vi "PI Receive String.vi"(0 "System no.":i32=1 min=1 step=1, 3 "Strip spaces?":bool, 5 "error in":errorcluster) -> (14 "String read":string, 15 "bytes read":u16, 19 "error out":errorcluster)   [LabVIEW 2026]
doc: "Read string from selected system."
uses:
  Available interfaces.ctl
  Available DLLs.ctl
  Available DLL interfaces.ctl
  Termination character.ctl
  Syntax.ctl
  Global1.vi
panel:
  out "Logging mode":bool
  out "Syntax":T1
  out "Termination character":T2
  out "VISA resource name":refnum<visa-resource-name>
  out "TCP/IP\nConfiguration":T3={"Host address/name"="localhost", "Port"=0, "Board"=4}
  out "DLL Interface Configuration":T6 {"DLL for Device" items=["C-843", "C-844", "E-710", "C-843.PM", "C-865", "E-761", "Mercury", "E-755", "E-753", "C-866", "E-712", "E-725", "E-861", "C-867", "E-517", "E-816", "E-709", "PI_GCS2_DLL", "HydraPollux"]; "DLL Interface" items=["RS232", "GPIB", "Board", "TCP-IP", "USB", "RS232_DC"]}
  out "Interface configuration":T8={"RS232 Portnumber"=0, "Timeout"=5000, "RS232 baud rate"=57600, "Interface"=0, "GPIB Bus"=0, "GPIB address"=4, "GPIB Mode"=0} {"Interface" items=["RS232", "GPIB", "DLL", "TCP-IP", "USB", "Analog"]; "RS232 Portnumber" items=["COM1", "COM2", "COM3", "COM4", "COM5", "COM6", "COM7", "COM8", "COM9", "COM10", "COM11", "COM12", "COM13", "COM14", "COM15", "COM16", "COM17", "COM18", "COM19", "COM20", "COM21", "COM22", "COM23", "COM24", "COM25", "COM26", "COM27", "COM28", "COM29", "COM30"]}
  # "This vi receives a string via the selected interface."
  # "Communication setup indicators (for troubleshooting):"
  # "TCP/IP:"
  # "DLL:"
  # "General:"
  # "RS232:"
  # "GPIB:"
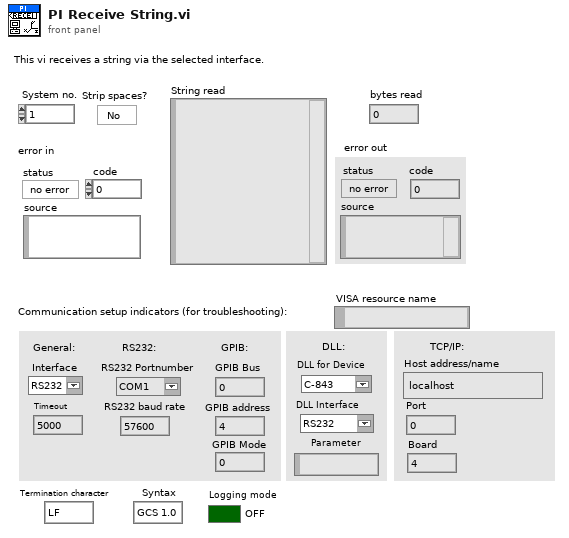
[diagram p1: front panel]
types:
  T1 = typedef "Syntax.ctl" = enum16{"GCS 1.0", "GCS 2.0", "GCS 3.0"}
  T2 = typedef "Termination character.ctl" = enum16{"LF", "CR", "LFCR", "CRLF"}
  T3 = cluster{"Host address/name":string, "Port":i32, "Board":i32}
  T4 = typedef "Available DLLs.ctl" = u16
  T5 = typedef "Available DLL interfaces.ctl" = u16
  T6 = cluster{"DLL for Device":T4, "DLL Interface":T5, "Parameter":string}
  T7 = typedef "Available interfaces.ctl" = u16
  T8 = cluster{"RS232 Portnumber":i32, "Timeout":i32, "RS232 baud rate":u32, "Interface":T7, "GPIB Bus":i32, "GPIB address":i32, "GPIB Mode":i32}
  T9 = cluster{"DLL for Device":T4, "DLL Interface":T5, "Parameter":string}[]
  T10 = cluster{"RS232 Portnumber":i32, "Timeout":i32, "RS232 Baud rate":u32, "Interface":T7, "GPIB Bus":i32, "GPIB Address":i32, "GPIB Mode":i32}[]
  T11 = cluster{"Host address/name":string, "Port":i32, "Board":i32}[]
  T12 = cluster{"RS232 Portnumber":i32, "Timeout":i32, "RS232 Baud rate":u32, "Interface":T7, "GPIB Bus":i32, "GPIB Address":i32, "GPIB Mode":i32}
  T13 = enum16{"C844_IsDLLAvailable", "C844_ConnectRS232", "C844_ConnectNIgpib", "C844_IsConnected", "C844_CloseConnection", "C844_GcsCommandset", "C844_GetError", "C844_GcsGetAnswerSize", "C844_GcsGetAnswer", "C843_IsDLLAvailable", "C843_Connect", "C843_IsConnected", "C843_CloseConnection", "C843_GcsCommandset", "C843_GetError", "C843_GcsGetAnswerSize", "C843_GcsGetAnswer", "E710_IsDLLAvailable", "E710_ConnectRS232", "E710_ConnectNIgpib", "E710_IsConnected", "E710_CloseConnection", "E710_GcsCommandset", "E710_GetError", "E710_GcsGetAnswerSize", "E710_GcsGetAnswer", "C843_PM_IsDLLAvailable", "C843_PM_Connect", "C843_PM_IsConnected", "C843_PM_CloseConnection", "C843_PM_GcsCommandset", "C843_PM_GetError", "C843_PM_GcsGetAnswerSize", "C843_PM_GcsGetAnswer", "C843_PM_GetCurrentBoardID", "C843_GetCurrentBoardID", "C865_IsDLLAvailable", "C865_ConnectRS232", "C865_IsConnected", "C865_CloseConnection", "C865_GcsCommandset", "C865_GetError", "C865_GcsGetAnswerSize", "C865_GcsGetAnswer", "C865_GetCurrentInterfaceID", "E761_ConnectPciBoard", "DefineSystem", "CloseConnection", "IsConnected", "ConnectRS232", "ConnectNIgpib", "ConnectPciBoard", "ConnectTCPIP", "GetError", "GcsCommandset", "GCSGetAnswerSize", "GcsGetAnswer", "CloseDaisyChain", "OpenRS232DaisyChain", "ConnectDaisyChainDevice", "ConnectUSB", "ListUSB", "OpenUSBDaisyChain", "OpenTCPIPDaisyChain"}
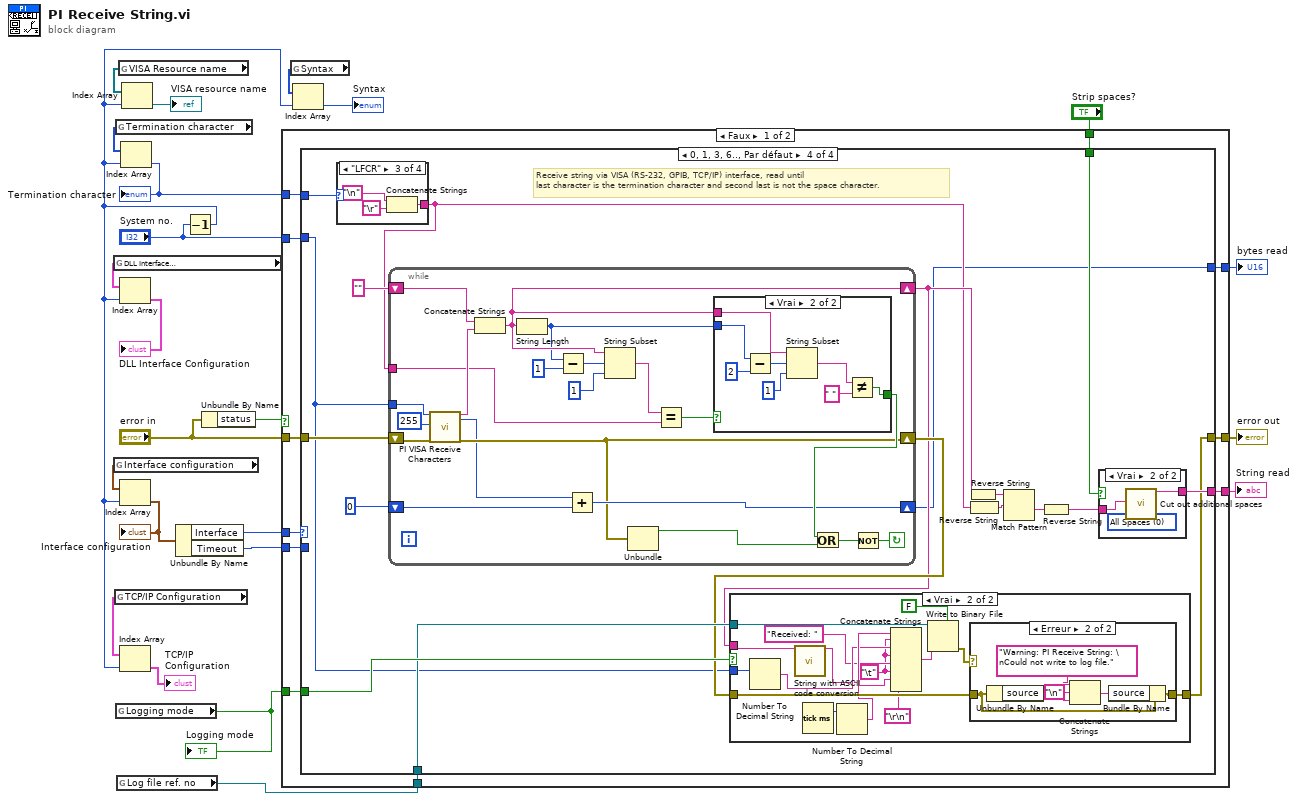
[diagram p0: block diagram]
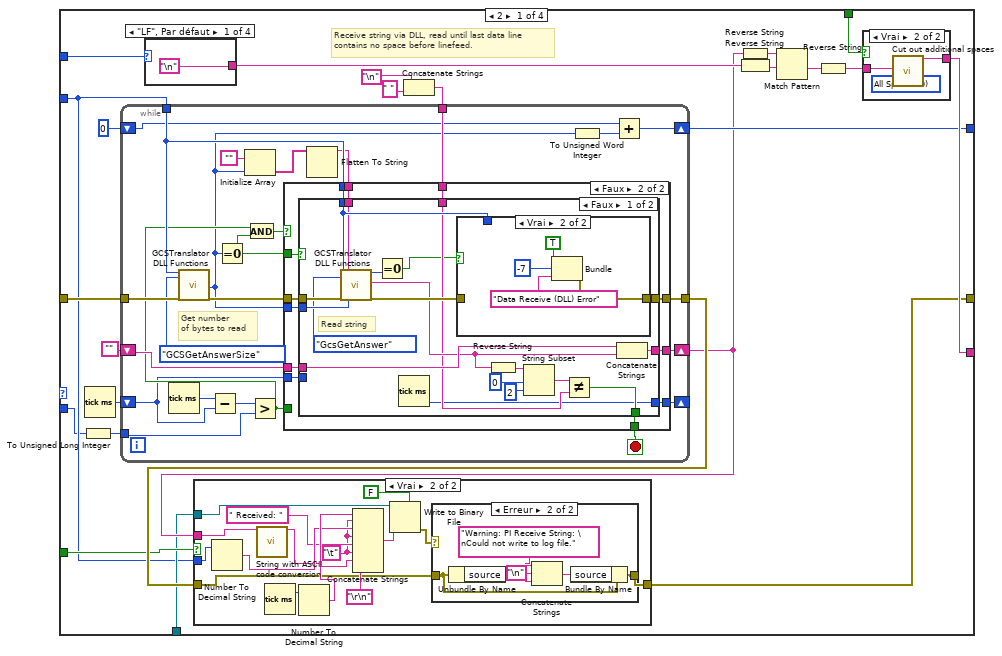
[diagram p2: hidden frame]
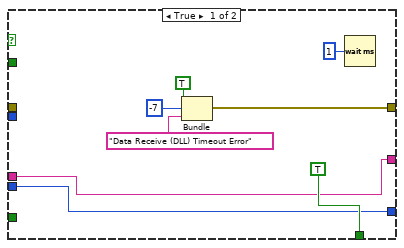
[diagram p5: hidden frame]
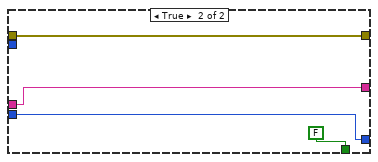
[diagram p7: hidden frame]
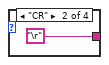
[diagram p8: hidden frame]
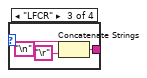
[diagram p9: hidden frame]
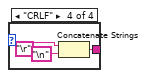
[diagram p10: hidden frame]
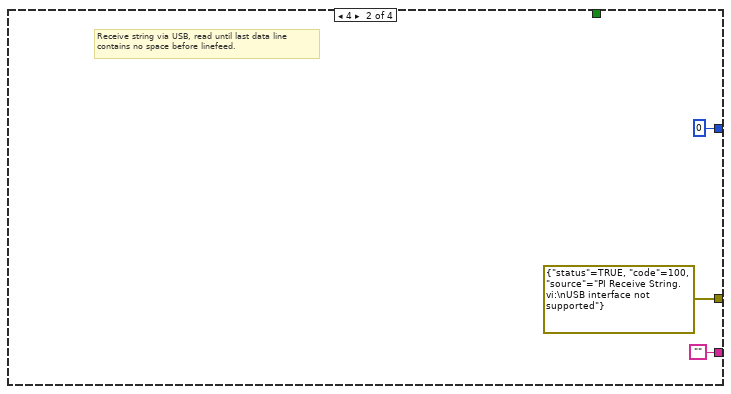
[diagram p12: hidden frame]
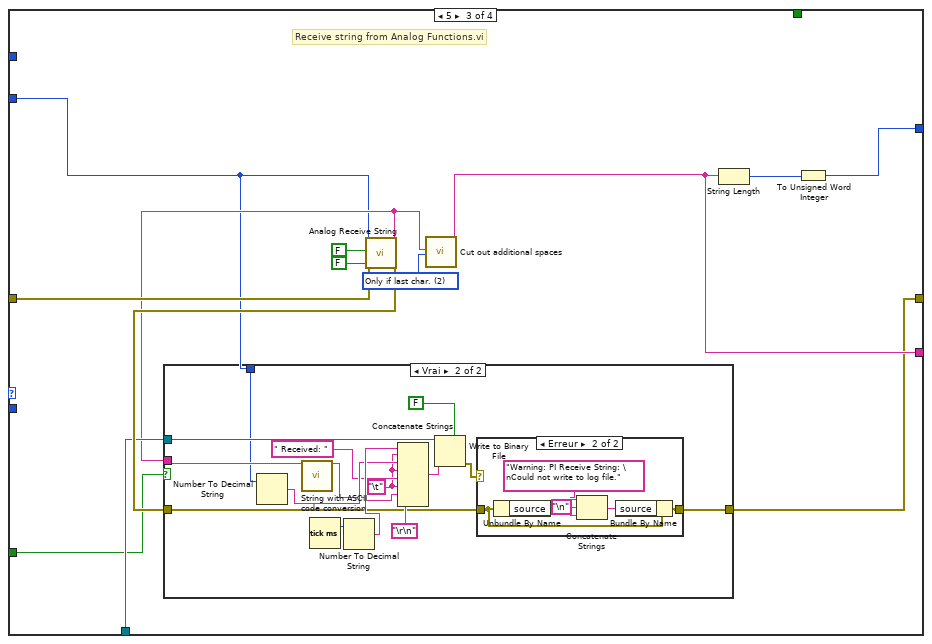
[diagram p13: hidden frame]
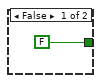
[diagram p16: hidden frame]
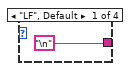
[diagram p20: hidden frame]
diagram:
  n1 = global read "Global1.vi" "DLL Interface\nConfiguration"() -> (w16:T9)
  n2 = global read "Global1.vi" "Interface configuration"() -> (w21:T10)
  n3 = global read "Global1.vi" "TCP/IP Configuration"() -> (w11:T11)
  n4 = global read "Global1.vi" "Termination character"() -> (w9:T2[])
  n5 = global read "Global1.vi" "Logging mode"() -> (w2:bool)
  "Logging mode" <- w2
  n6 = global read "Global1.vi" "Log file ref. no"() -> (w1:refnum<file>)
  n7 = global read "Global1.vi" "VISA Resource name"() -> (w13:refnum<visa-resource-name>[])
  n8 = Decrement(x="System no.") -> (x-1=w3:i32)
  n9 = Index Array(array=w16, index=w3) -> (element=→"DLL Interface Configuration":T6)
  n10 = Index Array(array=w21, index=w3) -> (element=w14:T12)
  "Interface configuration" <- w14
  n11 = Index Array(array=w11, index=w3) -> (element=→"TCP/IP\nConfiguration":T3)
  n12 = Index Array(array=w9, index=w3) -> (element=w8:T2)
  "Termination character" <- w8
  n13 = Index Array(array=w13, index=w3) -> (element=→"VISA resource name":refnum<visa-resource-name>)
  n14 = Unbundle By Name(w14) -> ("Interface"=w17:T7, "Timeout"=w4:i32)
  n15 = Unbundle By Name("error in") -> ("status"=w18:bool)
  n16 = case shown="Faux" w18 {
    tunnel: [w35 "" ("String read")] -> w24
    tunnel: "error in" -> [w34 w289]
    tunnel: w17 -> [w33 _]
    tunnel: [w32 u16 0 ("Bytes read")] -> w23
    tunnel: [w31 w289] -> w22
    tunnel: "System no." -> [w30 _]
    tunnel: w8 -> [w29 _]
    tunnel: "Strip spaces?" -> [w28 _]
    tunnel: w4 -> [w27 _]
    tunnel: w2 -> [w26 _]
    tunnel: w1 -> [w25 _]
    frame False {
      n17 = case shown="0, 1, 3, 6.., Par défaut" w33 {
        tunnel: [w58 "" ("String out") w181 w218] -> w35
        tunnel: w34 -> [w59 _ w178 w213]
        tunnel: [w50 u16 0 w170 w207] -> w32
        tunnel: [w39 errorcluster {"status"=TRUE, "code"=100, "source"="PI Receive String.vi:\nUSB interface not supported"} w176 w214] -> w31
        tunnel: w30 -> [w38 _ w172 w208]
        tunnel: w29 -> [w53 _ _ w223]
        tunnel: w28 -> [w57 _ _ w217]
        tunnel: w27 -> [w36 _ _ _]
        tunnel: w26 -> [w41 _ w174 w216]
        tunnel: w25 -> [w40 _ w175 w215]
        frame 2 {
          # "Receive string via DLL, read until last data line\ncontains no space before linefeed."
          n18 = To Unsigned Long Integer(number=w36) -> (unsigned 32bit integer=w37:u32)
          n19 = Tick Count (ms)() -> (millisecond timer value=w44:u32)
          n20 = case shown="\"LF\", Par défaut" w53 {
            tunnel: ["\n" "\r" w157 w162] -> w52
            frame "LF", Default {
            }
            frame "CR" {
            }
            frame "LFCR" {
              n21 = Concatenate Strings("\n", "\r") -> (w157:string)
            }
            frame "CRLF" {
              n22 = Concatenate Strings("\r", "\n") -> (w162:string)
            }
          }
          n23 = Concatenate Strings("\n", " " ("string")) -> (w47:string)
          n24 = while {
            tunnel: w59 -> [w106]
            tunnel: [w105] -> w43
            tunnel: w38 -> [w104]
            shift-right: [w98] -> w42
            shift-left: "" -> [w97]
            tunnel: w47 -> [w96]
            tunnel: w37 -> [w83]
            shift-right: [w89] -> _
            shift-left: w44 -> [w88]
            shift-right: [w99] -> w50
            shift-left: u16 0 -> [w86]
            stop <- w95 stop-if-true
            # "Get number\nof bytes to read"
            n25 = Tick Count (ms)() -> (millisecond timer value=w93:u32)
            n26 = call "GCSTranslator DLL Functions.vi"("System no."=w104, "Function"=T13."GCSGetAnswerSize", "error in"=w106) -> ("Numerical output"=w84:i32, "error out"=w100:errorcluster)  [unwired: 4 in, 11 out]
            n27 = Subtract(x=w93, y=w88) -> (x-y=w92:u32)
            n28 = Equal To 0?(x=w84) -> (x = 0?=w90:bool)
            n29 = Initialize Array("", w84) -> (w102:string[])
            n30 = Greater?(x=w92, y=w83) -> (0:w91:bool)
            n31 = And(x=w91, y=w90) -> (x .and. y?=w94:bool)
            n32 = Flatten To String(anything=w102) -> (data string=w101:string)  [unwired: 1 in, 4 out]
            n33 = case shown="Faux" w94 {
              tunnel: [w114 w126] -> w105
              tunnel: w104 -> [_ w125]
              tunnel: w101 -> [_ w124]
              tunnel: w100 -> [_ w123]
              tunnel: w84 -> [_ w122]
              tunnel: [w111 w121] -> w98
              tunnel: w97 -> [w111 w120]
              tunnel: w96 -> [_ w119]
              tunnel: [TRUE w118] -> w95
              tunnel: w91 -> [_ _]
              tunnel: w90 -> [_ w116]
              tunnel: [w110 w117] -> w89
              tunnel: w88 -> [w110 w115]
              frame True {
                n34 = Bundle(TRUE, -7, "Data Receive (DLL) Timeout Error") -> (w114:errorcluster)  [unwired: 1 out]
                n35 = Wait (ms)(milliseconds to wait=u32 1) -> ()  [unwired: 1 out]
              }
              frame False {
                n36 = case shown="Faux" w116 {
                  tunnel: [w145 w154] -> w126
                  tunnel: w125 -> [w144 _]
                  tunnel: w124 -> [w143 _]
                  tunnel: w123 -> [w142 w154]
                  tunnel: w122 -> [w139 _]
                  tunnel: [w138 w153] -> w121
                  tunnel: w120 -> [w137 w153]
                  tunnel: w119 -> [w132 _]
                  tunnel: [w131 FALSE] -> w118
                  tunnel: [w128 w152] -> w117
                  tunnel: w115 -> [_ w152]
                  frame False {
                    # "Read string"
                    n37 = call "GCSTranslator DLL Functions.vi"("System no."=w144, "Function"=T13."GcsGetAnswer", "error in"=w142, "String buffer"=w143, "Numerical input"=w139) -> ("DLL I32 Return value"=w141:i32, "String output"=w136:string, "error out"=w140:errorcluster)  [unwired: 2 in, 10 out]
                    n38 = Equal To 0?(x=w141) -> (x = 0?=w129:bool)
                    n39 = Tick Count (ms)() -> (millisecond timer value=w128:u32)
                    n40 = case shown="Vrai" w129 {
                      tunnel: [w146 w148] -> w145
                      tunnel: w144 -> [_ _]
                      tunnel: w140 -> [w146 _]
                      frame False {
                        # "no error"
                      }
                      frame True {
                        n41 = Bundle(TRUE, -7, "Data Receive (DLL) Error") -> (w148:errorcluster)  [unwired: 1 out]
                      }
                    }
                    n42 = Reverse String(1:w136) -> (0:w135:string)
                    n43 = String Subset(string=w135, offset (0)=0, length (rest)=2 ("length (rest)")) -> (substring=w133:string)
                    n44 = Not Equal?(x=w133, y=w132) -> (x != y?=w131:bool)
                    n45 = Concatenate Strings(w137, w136) -> (w138:string)
                  }
                  frame True {
                  }
                }
              }
            }
            n46 = To Unsigned Word Integer(number=w84) -> (unsigned 16bit integer=w85:u16)
            n47 = Add(x=w86, y=w85) -> (x+y=w99:u16)
          }
          n48 = case shown="Vrai" w41 {
            tunnel: w40 -> [_ w64]
            tunnel: w42 -> [_ w63]
            tunnel: w43 -> [w60 w65]
            tunnel: [w60 w66] -> w39
            tunnel: w38 -> [_ w62]
            frame False {
            }
            frame True {
              w69 = "\t"
              n49 = Number To Decimal String(number=w62) -> (decimal integer string=w71:string)  [unwired: 1 out]
              n50 = call "String with ASCII code conversion.vi"("Input string"=w63) -> ("Output string"=w68:string)  [unwired: 18 out]
              n51 = Tick Count (ms)() -> (millisecond timer value=w73:u32)
              n52 = Number To Decimal String(number=w73) -> (decimal integer string=w72:string)  [unwired: 1 out]
              n53 = Concatenate Strings(w72, w69, w71, w69, " Received: " ("string"), w69, w68, "\r\n") -> (w75:string)
              n54 = Write to Binary File(file (use dialog)=w64, data=w75, 5:FALSE ("prepend array or string size? (T)")) -> (error out=w74:errorcluster)  [unwired: 1 in, 4 out]
              n55 = case shown="Erreur" w74 {
                tunnel: w65 -> [w76 w82]
                tunnel: [w76 w78] -> w66
                frame No Error {
                }
                frame Error {
                  n56 = Unbundle By Name(w82) -> ("source"=w81:string)
                  n57 = Concatenate Strings(w81, "\n" ("string"), "Warning: PI Receive String: \nCould not write to log file." ("source")) -> (w77:string)
                  n58 = Bundle By Name(cluster=w82, "source"=w77) -> (w78:errorcluster)
                }
              }
            }
          }
          n59 = Reverse String(1:w42) -> (0:w55:string)
          n60 = Reverse String(1:w52) -> (0:w54:string)
          n61 = Match Pattern(string=w55, regular expression=w54) -> (after substring=w56:string)  [unwired: 4 out]
          n62 = Reverse String(1:w56) -> (0:w51:string)
          n63 = case shown="Vrai" w57 {
            tunnel: w51 -> [w163 w166]
            tunnel: [w163 w165] -> w58
            frame False {
            }
            frame True {
              w164 = u16 0 items=["All Spaces", "Only if 1st char.", "Only if last char.", "Only if near \"=\"", "Only if 1st or last char.", "Only multiple"] ("Mode")
              n64 = call "Cut out additional spaces.vi"("String"=w166, "Mode"=w164) -> ("String out"=w165:string)  [unwired: 17 out]
            }
          }
        }
        frame 4 {
          # "Receive string via USB, read until last data line\ncontains no space before linefeed."
        }
        frame 5 {
          w182 = u16 2 items=["All Spaces", "Only if 1st char.", "Only if last char.", "Only if near \"=\"", "Only if 1st or last char.", "Only multiple"] ("Mode")
          # "Receive string from Analog Functions.vi"
          n65 = call "Analog Receive String.vi"("System no."=w172, "Read/Write (T)"=FALSE, "Ini"=FALSE, "error in"=w178) -> ("String out"=w173:string, "error out"=w177:errorcluster)  [unwired: 1 in, 13 out]
          n66 = case shown="Vrai" w174 {
            tunnel: w175 -> [_ w189]
            tunnel: w173 -> [_ w188]
            tunnel: w177 -> [w183 w187]
            tunnel: [w183 w186] -> w176
            tunnel: w172 -> [_ w185]
            frame False {
            }
            frame True {
              w192 = "\t"
              n67 = Number To Decimal String(number=w185) -> (decimal integer string=w194:string)  [unwired: 1 out]
              n68 = call "String with ASCII code conversion.vi"("Input string"=w188) -> ("Output string"=w191:string)  [unwired: 18 out]
              n69 = Tick Count (ms)() -> (millisecond timer value=w196:u32)
              n70 = Number To Decimal String(number=w196) -> (decimal integer string=w195:string)  [unwired: 1 out]
              n71 = Concatenate Strings(w195, w192, w194, w192, " Received: " ("string"), w192, w191, "\r\n") -> (w198:string)
              n72 = Write to Binary File(file (use dialog)=w189, data=w198, 5:FALSE ("prepend array or string size? (T)")) -> (error out=w197:errorcluster)  [unwired: 1 in, 4 out]
              n73 = case shown="Erreur" w197 {
                tunnel: w187 -> [w199 w205]
                tunnel: [w199 w201] -> w186
                frame No Error {
                }
                frame Error {
                  n74 = Unbundle By Name(w205) -> ("source"=w204:string)
                  n75 = Concatenate Strings(w204, "\n" ("string"), "Warning: PI Receive String: \nCould not write to log file." ("source")) -> (w200:string)
                  n76 = Bundle By Name(cluster=w205, "source"=w200) -> (w201:errorcluster)
                }
              }
            }
          }
          n77 = call "Cut out additional spaces.vi"("String"=w173, "Mode"=w182) -> ("String out"=w181:string)  [unwired: 17 out]
          n78 = String Length(string=w181) -> (length=w171:i32)
          n79 = To Unsigned Word Integer(number=w171) -> (unsigned 16bit integer=w170:u16)
        }
        frame 0, 1, 3, 6.., Default {
          # "Receive string via VISA (RS-232, GPIB, TCP/IP) interface, read until \nlast character is the termination character and second last is not the space character."
          n80 = case shown="\"LFCR\"" w223 {
            tunnel: ["\n" "\r" w283 w288] -> w209
            frame "LF", Default {
            }
            frame "CR" {
            }
            frame "LFCR" {
              n81 = Concatenate Strings("\n", "\r") -> (w283:string)
            }
            frame "CRLF" {
              n82 = Concatenate Strings("\r", "\n") -> (w288:string)
            }
          }
          n83 = while {
            shift-left: w213 -> [w237]
            shift-right: [w236] -> w212
            tunnel: w208 -> [w235]
            shift-left: u16 0 -> [w239]
            shift-right: [w238] -> w207
            shift-left: "" -> [w244]
            shift-right: [w225] -> w211
            tunnel: w209 -> [w227]
            stop <- w241 continue-if-true
            n84 = call "PI VISA Receive Characters.vi"("System no."=w235, "Bytes to read"=u16 255, "error in"=w237) -> ("String read"=w232:string, "Bytes read"=w233:u16, "error out"=w236:errorcluster)  [unwired: 14 out]
            n85 = Concatenate Strings(w244, w232) -> (w225:string)
            n86 = String Length(string=w225) -> (length=w224:i32)
            n87 = Subtract(x=w224, y=1) -> (x-y=w230:i32)
            n88 = Add(x=w233, y=w239) -> (x+y=w238:u16)
            n89 = String Subset(string=w225, offset (0)=w230, length (rest)=1 ("length (rest)")) -> (substring=w228:string)
            n90 = Unbundle(w236) -> ("status"=w243:bool)  [unwired: 2 out]
            n91 = Equal?(x=w228, y=w227) -> (x = y?=w226:bool)
            n92 = case shown="Vrai" w226 {
              tunnel: [FALSE w252] -> w240
              tunnel: w225 -> [_ w250]
              tunnel: w224 -> [_ w246]
              frame False {
              }
              frame True {
                n93 = Subtract(x=w246, y=2) -> (x-y=w247:i32)
                n94 = String Subset(string=w250, offset (0)=w247, length (rest)=1 ("length (rest)")) -> (substring=w249:string)
                n95 = Not Equal?(x=w249, y=" ") -> (x != y?=w252:bool)
              }
            }
            n96 = Or(x=w240, y=w243) -> (x .or. y?=w242:bool)
            n97 = Not(x=w242) -> (.not. x?=w241:bool)
          }
          n98 = case shown="Vrai" w216 {
            tunnel: w215 -> [_ w269]
            tunnel: w211 -> [_ w264]
            tunnel: w212 -> [w254 w266]
            tunnel: [w254 w265] -> w214
            tunnel: w208 -> [_ w263]
            frame False {
            }
            frame True {
              w258 = "\t"
              n99 = Number To Decimal String(number=w263) -> (decimal integer string=w260:string)  [unwired: 1 out]
              n100 = call "String with ASCII code conversion.vi"("Input string"=w264) -> ("Output string"=w257:string)  [unwired: 18 out]
              n101 = Tick Count (ms)() -> (millisecond timer value=w262:u32)
              n102 = Number To Decimal String(number=w262) -> (decimal integer string=w261:string)  [unwired: 1 out]
              n103 = Concatenate Strings(w261, w258, w260, w258, "Received: " ("string"), w258, w257, "\r\n") -> (w268:string)
              n104 = Write to Binary File(file (use dialog)=w269, data=w268, 5:FALSE ("prepend array or string size? (T)")) -> (error out=w267:errorcluster)  [unwired: 1 in, 4 out]
              n105 = case shown="Erreur" w267 {
                tunnel: w266 -> [w270 w276]
                tunnel: [w270 w272] -> w265
                frame No Error {
                }
                frame Error {
                  n106 = Unbundle By Name(w276) -> ("source"=w275:string)
                  n107 = Concatenate Strings(w275, "\n" ("string"), "Warning: PI Receive String: \nCould not write to log file." ("source")) -> (w271:string)
                  n108 = Bundle By Name(cluster=w276, "source"=w271) -> (w272:errorcluster)
                }
              }
            }
          }
          n109 = Reverse String(1:w211) -> (0:w221:string)
          n110 = Reverse String(1:w209) -> (0:w220:string)
          n111 = Match Pattern(string=w221, regular expression=w220) -> (after substring=w222:string)  [unwired: 4 out]
          n112 = Reverse String(1:w222) -> (0:w219:string)
          n113 = case shown="Vrai" w217 {
            tunnel: w219 -> [w277 w280]
            tunnel: [w277 w279] -> w218
            frame False {
            }
            frame True {
              w278 = u16 0 items=["All Spaces", "Only if 1st char.", "Only if last char.", "Only if near \"=\"", "Only if 1st or last char.", "Only multiple"] ("Mode")
              n114 = call "Cut out additional spaces.vi"("String"=w280, "Mode"=w278) -> ("String out"=w279:string)  [unwired: 17 out]
            }
          }
        }
      }
    }
    frame True {
      # "Error!"
    }
  }
  "String read" <- w24
  "bytes read" <- w23
  "error out" <- w22
  n115 = global read "Global1.vi" "Syntax"() -> (w6:T1[])
  n116 = Index Array(array=w6, index=w3) -> (element=→"Syntax":T1)
